vi "Calculate Distance.vi"(0 "X1":sgl, 1 "Y1":sgl, 2 "X2":sgl, 3 "Y2":sgl) -> (7 "Distance":sgl)   [LabVIEW 2018]
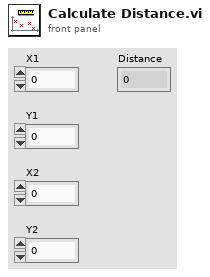
[diagram p1: front panel]
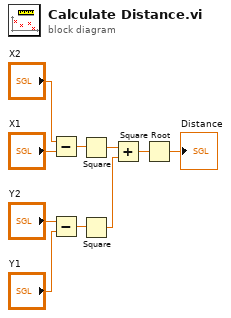
[diagram p0: block diagram]
diagram:
  n1 = Subtract(x="X2", y="X1") -> (x-y=w3:sgl)
  n2 = Subtract(x="Y2", y="Y1") -> (x-y=w4:sgl)
  n3 = Square(x=w3) -> (x^2=w5:sgl)
  n4 = Square(x=w4) -> (x^2=w6:sgl)
  n5 = Add(x=w5, y=w6) -> (x+y=w7:sgl)
  n6 = Square Root(x=w7) -> (sqrt(x)=→"Distance":sgl)
